vi "AutoCal.vi"() -> (0 "Autocal mode?":bool)   [LabVIEW 2017, in "GP22_TDC_Arduinoed.lvlib"]
doc: "Check the current state of the registers to see if autocal mode is enabled."
uses:
  GP22_TDC_Arduinoed.lvlib
  Public/Globals.vi
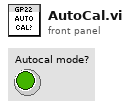
[diagram p1: front panel]
types:
  T1 = typedef "GP22_TDC_Arduinoed.lvlib/Registers.ctl" = cluster{"Reg0":u32, "Reg1":u32, "Reg2":u32, "Reg3":u32, "Reg4":u32, "Reg5":u32, "Reg6":u32}
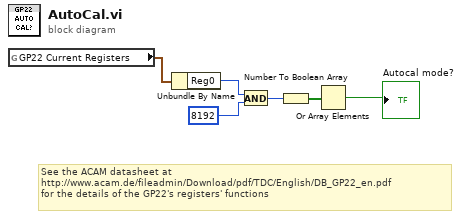
[diagram p0: block diagram]
diagram:
  # "See the ACAM datasheet at \nhttp://www.acam.de/fileadmin/Download/pdf/TDC/English/DB_GP22_en.pdf\nfor the details of the GP22's registers' functions"
  n1 = global read "Globals.vi" "GP22 Current Registers"() -> (w6:T1)
  n2 = Unbundle By Name(w6) -> ("Reg0"=w5:u32)
  n3 = And(x=w5, y=u32 8192 ("Reg0")) -> (x .and. y?=w3:u32)
  n4 = Number To Boolean Array(number=w3) -> (Boolean array=w2:bool[])
  n5 = Or Array Elements(Boolean array=w2) -> (logical OR=→"Autocal mode?":bool)
